vi "refresh C1 duty cycle.vi"(8 "error in (no error)":errorcluster, 11 "Waveform in":refnum<class "Waveform.lvclass">) -> (0 "error out":errorcluster, 3 "Waveform out":refnum<class "Waveform.lvclass">)   [LabVIEW 2012, in "Waveform.lvclass"]
uses:
  Waveform.lvclass
  Waveform.lvclass/Waveform.ctl
  <resource>/objmgr/daqmx.rc
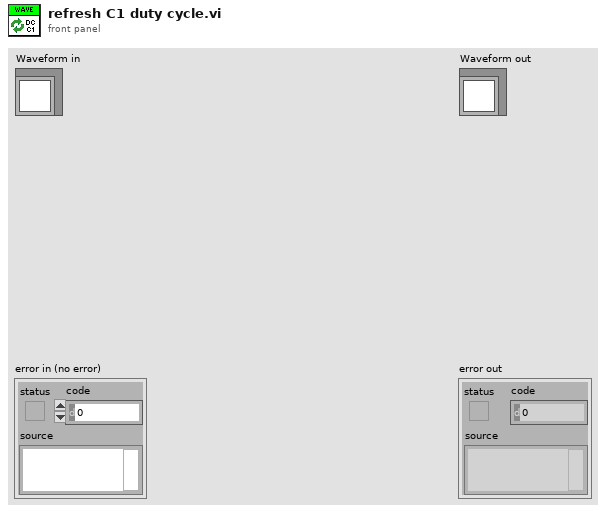
[diagram p1: front panel]
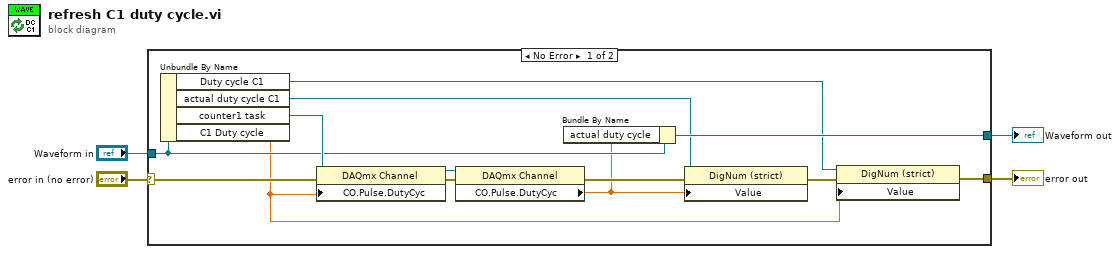
[diagram p0: block diagram]
diagram:
  n1 = case shown="No Error" "error in (no error)" {
    selector: "error in (no error)" -> [w9 w19]
    tunnel: [w8 w19] -> w3
    tunnel: [w12 w18] -> w1
    tunnel: "Waveform in" -> [w13 w18]
    frame No Error {
      n2 = Unbundle By Name(w13) -> ("Duty cycle C1"=w6:refnum<vi>, "actual duty cycle C1"=w11:refnum<vi>, "counter1 task"=w14:refnum<k21>, "C1 Duty cycle"=w5:dbl)
      n3 = property class="DAQmx Channel"(reference=w14, error in=w9, "CO.Pulse.DutyCyc"=w5) -> (reference out=w15:refnum<k21>, error out=w16:errorcluster)
      n4 = property class="DAQmx Channel"(reference=w15, error in=w16) -> (error out=w17:errorcluster, "CO.Pulse.DutyCyc"=w10:dbl)  [unwired: 1 out]
      n5 = Bundle By Name(cluster=w13, "actual duty cycle"=w10) -> (w12:refnum<class "Waveform.lvclass">)
      n6 = property class="DigNum (strict)"(reference=w11, error in=w17, "Value"=w10) -> (error out=w7:errorcluster)  [unwired: 1 out]
      n7 = property class="DigNum (strict)"(reference=w6, error in=w7, "Value"=w5) -> (error out=w8:errorcluster)  [unwired: 1 out]
    }
    frame Error {
    }
  }
  "error out" <- w3
  "Waveform out" <- w1
